vi "Reinitialize.vi"(8 "error in (no error)":errorcluster, 11 "MODBUS in":refnum<class "Modbus.lvclass">) -> (0 "error out":errorcluster, 3 "MODBUS Out":refnum<class "Modbus.lvclass">)   [LabVIEW 2020, in "Library Instrument & Equipement.lvlib" / "Library Relay_Board.lvlib" / "Modbus.lvclass"]
doc: "Reinitializes connection to Modbus server based on previously specified settings."
uses:
  Modbus.lvclass
  Modbus.lvclass/Modbus.ctl
  <vilib>/Instr/_visa.llb/VISA Configure Serial Port (Instr).vi
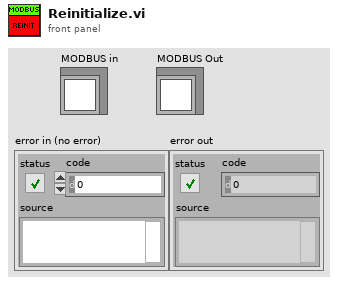
[diagram p1: front panel]
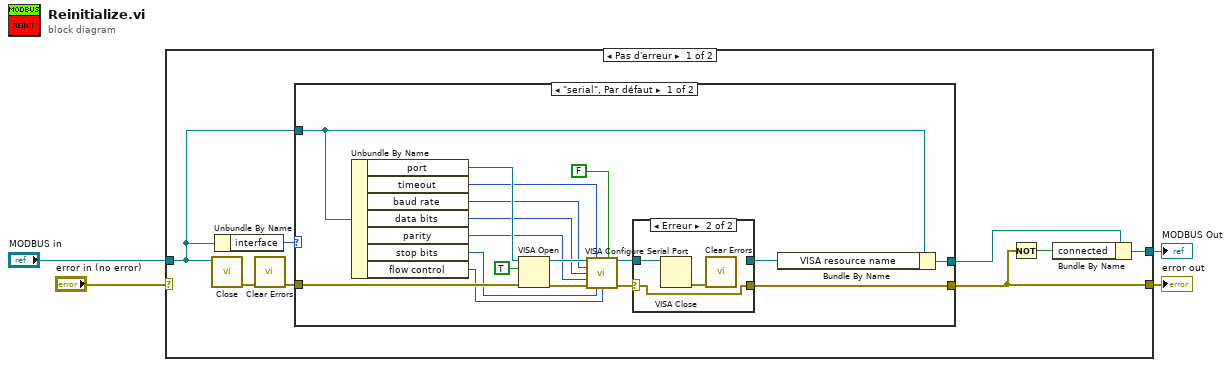
[diagram p0: block diagram]
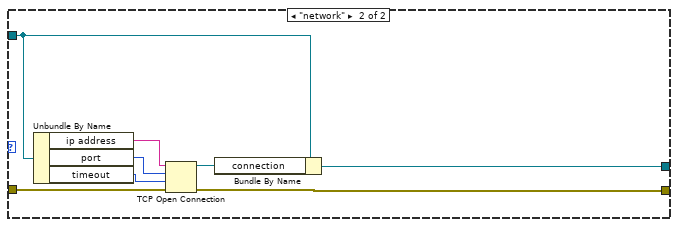
[diagram p3: hidden frame]
diagram:
  n1 = case shown="Pas d'erreur" "error in (no error)" {
    selector: "error in (no error)" -> [_ w44]
    tunnel: "MODBUS in" -> [w12 w45]
    tunnel: [w8 w45] -> w3
    tunnel: [w7 w44] -> w2
    frame No Error {
      n2 = call-dynamic "Close.vi"("MODBUS in"=w12) -> ("error out"=w6:errorcluster)  [unwired: 10 in]
      n3 = Unbundle By Name(w12) -> ("interface"=w11:enum16{"serial", "network"})
      n4 = call <vilib>:"Clear Errors.vi"("error in (no error)"=w6) -> ("error out"=w5:errorcluster)  [unwired: 5 in, 1 out]
      n5 = case shown="\"serial\", Par défaut" w11 {
        tunnel: [w13 w37] -> w7
        tunnel: [w30 w42] -> w10
        tunnel: w12 -> [w27 w41]
        tunnel: w5 -> [w28 w40]
        frame "serial", Default {
          n6 = Unbundle By Name(w27) -> ("port"=w26:refnum<visa-resource-name>, "timeout"=w20:u32, "baud rate"=w24:u32, "data bits"=w23:u16, "parity"=w22:enum16{"None", "Odd", "Even", "Mark", "Space"}, "stop bits"=w19:u16, "flow control"=w18:u16)
          n7 = VISA Open(duplicate session (F)=TRUE, error in (no error)=w28, VISA resource name=w26) -> (VISA resource name=w25:refnum<visa-resource-name>, error out=w21:errorcluster)  [unwired: 2 in]
          n8 = call-poly "VISA Configure Serial Port"("VISA resource name"=w25, "timeout (10sec)"=w20, "Enable Termination\nChar (T)"=FALSE ("Enable Termination\nChar (T)"), "baud rate (9600)"=w24, "data bits (8)"=w23, "parity (0:none)"=w22, "error in (no error)"=w21, "stop bits (10: 1 bit)"=w19, "flow control (0:none)"=w18) -> ("VISA resource name out"=w15:refnum<visa-resource-name>, "error out"=w16:errorcluster)  [unwired: 5 in]
          n9 = case shown="Erreur" w16 {
            selector: w16 -> [w31 w33]
            tunnel: w15 -> [w32 w35]
            tunnel: [w32 _] -> w14
            tunnel: [w31 w33] -> w13
            frame No Error {
            }
            frame Error {
              n10 = VISA Close(VISA resource name=w35) -> (error out=w34:errorcluster)  [unwired: 1 in]
              n11 = call <vilib>:"Clear Errors.vi"("error in (no error)"=w34) -> ()  [unwired: 5 in, 2 out]
            }
          }
          n12 = Bundle By Name(cluster=w27, "VISA resource name"=w14) -> (w30:refnum<class "Modbus.lvclass">)
        }
        frame "network" {
          n13 = Unbundle By Name(w41) -> ("ip address"=w36:string, "port"=w38:u16, "timeout"=w39:u32)
          n14 = TCP Open Connection(address=w36, remote port or service name=w38, timeout ms (60000)=w39, error in (no error)=w40) -> (connection ID=w43:refnum<k5>, error out=w37:errorcluster)  [unwired: 1 in]
          n15 = Bundle By Name(cluster=w41, "connection"=w43) -> (w42:refnum<class "Modbus.lvclass">)
        }
      }
      n16 = Not(x=w7) -> (.not. x?=w9:bool)
      n17 = Bundle By Name(cluster=w10, "connected"=w9) -> (w8:refnum<class "Modbus.lvclass">)
    }
    frame Error {
    }
  }
  "MODBUS Out" <- w3
  "error out" <- w2
